vi "L00.vi"() -> ()   [LabVIEW 2012]
panel:
  in  "Array 4":u16[](array[ring])
  in  "Array 3":u16[](array[ring])
  in  "Array 2":u16[](array[ring])
  in  "Array":u16[](array[ring])
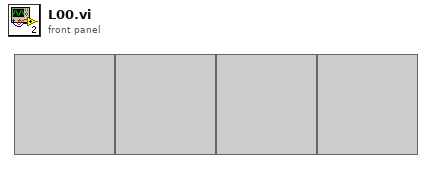
[diagram p1: front panel]
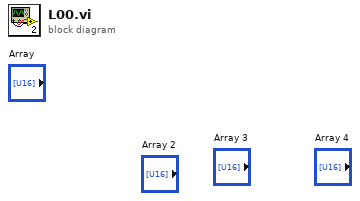
[diagram p0: block diagram]
diagram:
